vi "Ask Component and Tool ID.vi"(11 "Module In":refnum<class "Module.lvclass">) -> (3 "Module Out":refnum<class "Module.lvclass">)   [LabVIEW 2018, in "Module.lvclass"]
uses:
  Module.lvclass
  Module.lvclass/Module.ctl
panel:
  out "Module":string
  in  "Submit":bool
  in  "ID":i32
  in  "ID":i32
  out "Pick-Up Tool":string
  out "Component":string
  # "Component"
  # "Pick-Up Tool"
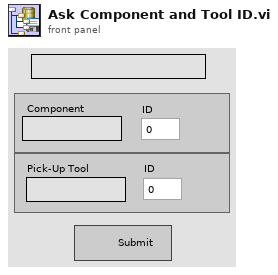
[diagram p1: front panel]
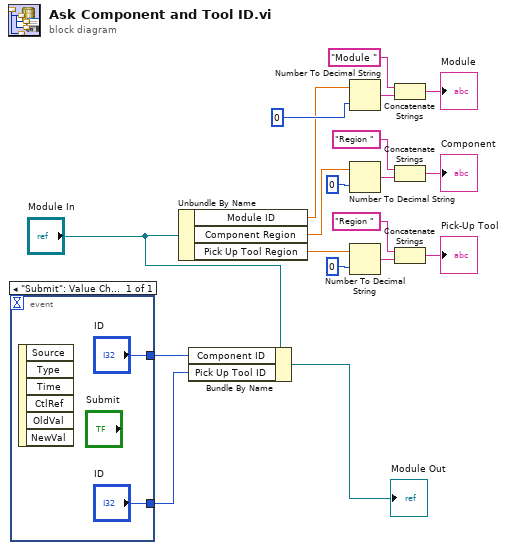
[diagram p0: block diagram]
diagram:
  n1 = event shown="[0] \"Submit\": Value Change" {
    selector: _ -> [_]
    dyn-events: _ -> [_]
    timeout: _ -> [_]
    tunnel: ["ID"] -> w7
    tunnel: ["ID"] -> w8
    event "Submit": Value Change {
      n2 = event-data() -> ()  [unwired: 1 in, 6 out]
    }
  }
  n3 = Unbundle By Name("Module In") -> ("Module ID"=w1:dbl, "Component Region"=w11:dbl, "Pick Up Tool Region"=w10:dbl)
  n4 = Bundle By Name(cluster="Module In", "Component ID"=w8, "Pick Up Tool ID"=w7) -> (→"Module Out":refnum<class "Module.lvclass">)
  n5 = Number To Decimal String(number=w1, width (-)=i16 0) -> (decimal integer string=w3:string)
  n6 = Number To Decimal String(number=w11, width (-)=i16 0) -> (decimal integer string=w15:string)
  n7 = Number To Decimal String(number=w10, width (-)=i16 0) -> (decimal integer string=w18:string)
  n8 = Concatenate Strings("Module ", w3) -> (→"Module":string)
  n9 = Concatenate Strings("Region ", w15) -> (→"Component":string)
  n10 = Concatenate Strings("Region ", w18) -> (→"Pick-Up Tool":string)
